vi "Day 8-1.vi"() -> ()   [LabVIEW 2019, in "Day 8.lvlib"]
uses:
  Day 8.lvlib
panel:
  out "Array":string[][](array[string])
  out "disabled index (col)":i32
  out "array type (2D Dbl)":string[][](array[string])
  out "subarray":string[](array[string])
  out "array":string[][](array[string])
  in  "String":string="ecgabfd gfbe dgbeaf aeg gfbda eg bgdcaf efgdca abced eadgb | begf decgfa aeg eg\nebfg bfgdea gaf gf baedgc dafec cfdabg ecfabgd fdgea dbaeg | gaedbc egbf dbgcea dagfebc\ncfadeg ca bacg dfabe dgcbf dbegafc dac afbdgc gcbedf bfcda | fbdac adbef bgcdfae dcagfe\neag cdgfae cbdge ae fcgad eabdfg ecaf gefbadc dgafcb degca | dacbefg fcdage agdcf fedagb\ndga edac gdfbea bgdfec da cfbga dbgec cadgb bdgace dcbfage | acgfb gaecbfd dag gedfab\ncefb fb abcgefd fagbde fcbgae faecg cbadg cbfga bfa agcdef | gbacf agbfc bgcaef baf\nebdacf cbgfae cgdebaf afdcb gabdc df cdf eafd ecabf begdfc | cbdaf gdabc fd cbefda\nge daebc fcagb fdebac gaed ecabg egc gacedb cbdfeg adcfbeg | gec gebdca ebagc adbgcfe\nbgfade gcefbd eafgd fcae cadgf gcf dgcba cfdega cagbdfe cf | cdgeaf agfed cf cf\nabfge ebac acfegbd bc fcged gbfec cfgbad fecabg agbfde fcb | aefgdb cfb egbfca cbfaedg\ndfcbag gda dcafe gcdeb ag ecgdaf edagc bcdaef gcbadfe gaef | gbced dga cbadef fgecda\ncagb adgceb cdb cfgeda egfbd abcefd decag bc cgebd bgedfca | cegbd dfegac dbc befdg\ncbfe bgefdc ceabdfg cf dbgaef gdfbac edcga gcfed dfc fbedg | fgbaed fcd fcegd becf\ndegabf bfg bcgaf gdacf dbfc gecfda gcaeb fagedbc adfgbc bf | egbdfa gbf adfbceg dcfb\ndbfae dfbc ecadg cb cbdea fcebag fgadbec gadebf bec ceabfd | dbfc bgfcead agbedf fdabe\ndafcge ecafbg cegaf egdac abegd cd debfca edc cgfd bfdeagc | dec dc ecd dbgae\nfgabce bfa acbfegd fcegda bfgd acgfd bcaed bfcda bf cbagdf | bf bafgcd bfdg dgbacfe\nfgea gad fcbgaed gdebc afdeb fagcbd cbfeda ag egfdba degab | dgeab badge eacfbdg fdceba\nfabdce cagdb gcb bcefag degba dfagbc dgcf dcfab egfcabd cg | befcda dbagc cbdgfa gcdf\nbe fgaced fdeag badegf fdbea ebdg bea agfbec ebgadcf bcfad | acdfge agbfce debaf dgafe\ncdfbeg bg fegca gdefac cadbf eadbcgf cgb egba gcfbea cagfb | gfaced agfcb cbdfaeg cgfdabe\nfadcebg cgda ebfag adebc fcebdg fadbce gd begcda bdg gedba | dcga fbage dcabef fcebadg\nbfcga adfbgc fbcdage gfedac ab gcfbe cgafd efabgd gab bdca | gcafd cdba gba dfabgc\nbdfae gfa cdgabe egfba fg gfeadc acegb fgcb fbecgad ecafgb | bgeaf agfecbd fga agdceb\ndgab ebfad cdefgb gbefd fab cefabg fegcbda aedcf ba ebadgf | defbag afb gbfead dbefag\ncfabed ecabf cgafdeb bfc fecbgd dcab cb bfeda eagfc adfgeb | fgcae dfbega ebcdfg fabec\neb cbgaef eagcfbd caebd gaedbc badfc abe degac dgeb cgdeaf | aeb gfaebc bceafg abcged\ngdecba ecbdgf def fcbade fd fdcg bgfae gdecb gfbde faegdbc | fbage ecgdbf egdfb dfe\ndc dac egcadbf gadbe cgaebd abgcd geadbf agfced edcb gabfc | agcbefd edbc bacfg cd\ngaebfc gdc cedbg dbeag cefd cd bcfgde cbgfda bcegf dabgecf | bgdea dbgec fecd cfed\nafd dfcbga dcbeagf bfecda egbcdf dagec fa bgfa fdbcg fgadc | egbcdf decga gbfa fa\nfg baefc gafeb dgaf cbgdea afegbd fbg cebgfd gaecdfb dbgae | ebfag dgbae gafd abgedfc\ncbaed gedac cefgbda feba be cadebf gdcefb fcbad bde cdagbf | bcadef cfgdab fdabc feab\ncfbdg fdgce adgcbf fb cbf acfegdb adgebc ebafdc dbacg agbf | fgba fgced ecfdabg bf\nfceabd gfb agfdb deabg beacgf cfdgbae fcdg gf abfdc dfbgca | dbaeg bfdga dgeab dfcg\ngfde facbde dcgbf fg gbf ecafgb cfgdbe ecdfb adcgb ecafbdg | gcdbf fg cfbdg fdeg\nfbgdce bg bacefg decab cbg fecgd egdcfa dbfg egdcb fagdbce | gb dcbea fedbgc fagecb\nabgcef fgbaedc dfaebg cgad ad egadcb abd cgbea bfecd cabde | efbcd abdfeg afbegd ad\nfagecdb bcafg ecadfb fa bagecf cdgba efbdcg befgc fac agfe | bdfcge ecgbf cfedba edagfcb\ndgf fcdbg cegbd fd bfcega daebgf dfca abgcf gafbdc fbeacgd | bcfdg fdg dfg adcf\ndeb cbdgae edfbac dbcgf fbecga gdfcbea bgdec ed ecabg egad | bgcfd faedcb cageb ed\ngecfba dfagc afdbc adbcfg cag cabgdfe fdega cbdg dbacfe cg | afcbdeg dabcf cbafed dcfga\nfeab ae cbgfe agecf bgecda bgecdf eca gfebca fcdbgea cgfad | bgdfec gcfbed eca cbdgaef\nfbaceg edcbaf dba becgd egafb degbfca fbadeg dafg da agebd | fbdega gfebca acebdf gbefa\ndbce gfbec defgb ed efdagc def gfbeca abfgd bgfedc fcbgade | fdbgce ebdfcg cgfbdea efcbgd\nabcdfg fcaegb egf dgcaf bdecf aged bdeacfg ge dgcafe gfcde | acbgfd gcadf cgbdaf gafecb\nfb gbfaed eabgdc abcgef adcbfge dgfac fecb bgf fcbga cageb | acebg cfeabg edgcab adgfbce\nfad ceafdg dcfag fbcadge geadbf deac da gcfea gdcfb efcagb | aegdfb cgadf aefbcg bgdcf\ndagcbf ef dacfg gfdce egf ebdgc dfcgea fabdeg aefc ebdacfg | gdefc dcfag bgdceaf acef\ndbegf eabcgd ebdafg fbdac cbg cefg eagbdfc cdbgf gdfbce cg | eabcdgf gecadbf decgbf gc\ndegf cbefd bfcdeg bfdaec bcage cfgdba fg fcg fbcge cefgdba | fged cfgedab fdgceb efcbd\ncgbdae dbeca bcfdeg fcaged edgca be cbdaf ebd gfbadec egba | cefdgab cdfega bcgeda agcbde\ncdfgea gbedacf gacbf cdb decag db edcabf gabedc dgeb bgdca | bcfag bcgad ecdgfab bd\nebcg cfgbae acgdbef eag agdfc ge edgabf cgefa facbe dacebf | cbgefa agcfd fgcad dfgac\nbeagcf dafcgbe da acd bedcf begacd cdbae cefadg bagd bgcae | da fgbecad bdcef bfdec\ndg acgfebd fagecb bgeadf ebfgc gdb cdbgf dbafc gecd debfgc | egcbf cafbd facbd afbegcd\ngeabd cadefb ec eadgfcb cedag gdbeca dec gfbdae dcfag cbeg | ec bdeafgc cbdafe ebcg\nbe bfade caefgb eab gdbafe bedg agfdb edacfbg gdcabf daefc | acfegb bae fecadgb bgcfea\nbe acdfb cgfae cbe agbe fgeacbd adegcf bcfae bgcefa fgbecd | cfabeg ecb efcdbg ageb\nafbg cfedb dacfgb fgdcb bgfedac cbdage bg acgdf fadceg dgb | cdbgfa fgeadc bafg dfbce\ndebfc efb adgbce ef fbadec dfcbg feac dacgebf aebdc eadgfb | fcdgb efca cbdeaf edbca\ngcbde dgcbf dfc bfcgda df ceadgbf gcabf dbaf gcefab dfcega | adfb egcdb dgbce bdfa\negbdca bgfed baefd cfdgaeb gdefc gcbfed gcfead bg cfgb egb | dcbage cbdgef dgfbe aedbcg\ndceaf fc fcge bgdaec agced dfbea cgeabdf adcfbg fdc egcfad | fedca fadeb dabegc aedfb\nacfbgd efcda cfagd decg de efcgdab eabfc gdaecf dae bedfag | fceda acdef ed cfeba\ndefbcg ge egb eagbdc afdgcb cgbae fcadebg geda dcagb efcba | gdecba abgce gbadc daeg\nafbd fadgce gbfdea fcgedb bf bgf gefda bfedgac bgcea gaebf | bgfaed fdgecb fbgedc bfg\ncbafgd cbdge bc cbd bcef fgbde afgbde fgcbed dgebfca edcga | cb cb acged fdgbec\nacgd dceagf dc bafde fbaceg ced cdfbge fdeca egcabfd cgefa | dc egdcfa afegcd efcgbd\nbgdfac fb aebgc bfde bdecaf bfa aebcf edabfcg cgdeaf daefc | decfa fb baf fcbdea\nbdfegc gebda gecbfa fedbg fed dgfc fabdec dbcagef fd gfcbe | edcfbag dgfeb cdeafb fd\ngbeadf fdcga ecadb bceg ge egd dgebacf beafcd aedgc cgbade | dabec dge begdac dgaebc\nbegc dcgbfa eb dfeag eafgb bae bcgaf gfaebc fbagecd becfad | gabdcfe fdcagb bgcdaf be\neca febdcg fedag ecdaf fcba beagdc fcdeb ca dbefca acebfdg | ebdcgf fdceb gecdab cedfbga\ndecfbga abgdce gefd afd aecdbf gcfeda acgde cafbg fd fadcg | edgf dafbceg egfd cedga\nfaedgbc fbgaec dacb eba geacdb bcgefd ba bdegc eadbg gdaef | dfcbge deabcg bfecadg gfcbaed\negfacbd acdgf gecdab ebacf abcfed eg begf caegf aeg bfgeca | dafbcge cadfg fbace cefdbag\ndgcfbae ac gbfeca badce gcad dfgcbe defab cea acgdbe dbgce | cgdeba egcdb gcad cagd\ndcfg agdfbc caedfgb df bagecf daf gcafb ebcad fdbac agebdf | bdfage fgdbac daf fd\nagefbd agcbfde egafb eg adge fge bfaced egdbcf daefb cabgf | bagef afgbe eg efbcdg\nadfegb caefgb ade ecgd cafed dbfeacg de fgcae fbcda fgadce | dbefgac eafcg gbaefc fedgac\ndbafg ecfga gfbae bae egdbac geabfc gcedfab ebcf eb cagdef | be cbfe bae be\ncfgadbe eca bcfadg ebdgac adgcb ebdca adbfe egcb cadfeg ec | adebgc feabd cae cgdfea\ncaefdg cdfagbe fadbc afd eacbd fd bcadeg cgfba dacfeb bfed | df afcgb fceabdg fda\nedcgaf cfbdag cbfdaeg ec cae bgeafc cdafe abfde decg gdcaf | eca dbcafg aec ce\nfbgae cagef egdbac cg gcdafbe cfbg bgefda gce ceadf gebfac | gadbce cdegba gc cg\nbafgecd bdf ecabfg dgbfe dcefg gbefa bdea bdfcga bd bgfdae | cdfagb cfeabg faebgd fagbe\nafg dfcg fg eacdbg fgadeb cfdgea ecagd fcagebd eacfg bacfe | fg dagecb egdca cfdg\ndac dc fgcd agbecf gcdaef agbed edcabf fgace caged faecdbg | dabge gceaf gdafecb cdafgeb\naefbg egf bagcf afegdc dfgceab begd gafebd eafbd eg fabcde | egadfb feg bgcfa efg\nfa debfg acgfdb eagbc dcebagf cedfbg dafe baf febga eagbfd | af cbfdga dcfgab befcdg\ndb dbfe fdbga cafdg adgceb egbfa dbg bgfdcea ceagbf befagd | afdbge dceabg gdfab fdaegb\nfgeacdb cadg dfg edfga fdagce dg dfaec gebfa cbefgd defabc | geabf dfaec cfdae faegb\nabdce bafcg gdecaf cegba fbcadge adbcfe degb eg bdcgae eag | abdec facbg edgb ebagcd\nbcaef fg dgbcae adegb bafeg feadcgb egbfad fdgb fecagd efg | agfeb fge fdgb eadgb\ndbfage cdab bgcaef ecb cb dgfce dfbce fedbgac deabf beadcf | cbfed dabfe ebadf cefbd\ngcedb ceafdg dcg gecdfb dcfaeb cg egdba befdgac fdceb gcfb | begdc bedag eadgb dfecb\nbf dbcgea eabdfc feb gbfeac fagb becga fcdaebg dcgef gecfb | efbdcag abceg gcdabef gcbef\nged dagfbe eg cgfe bgfacde gedac dceba agcfd cadegf gcfdba | gefc ge ge acegfbd\ngfabed aecdgf ecbag dge gbdae befd bfgad fdcabeg de fagbdc | egbad afdbg dgacef gdafb\ndabfegc gbcad gafd acd da fgbadc ecdabf bfgca fcabge gbdec | gbface fgcab bdgac ebdcg\nafbceg cdgfb gb afcbed dfcbge gbf adfgc fecbgad egdb bcdfe | fedbc cfeabd edbg cfebgd\ncbdae gc gdfc ebgdf gcafbe fbaecdg gbedc ecg fbgecd fdebag | gcedb ebgafc acfgdeb ceg\nbdce efacgd dgfbc ebfgad bcfga gdc fgbedac egdfb dc bfdgce | bagdfec efdgb ecbd fdaegc\nbdgefc fbca bc gfbcae fdcgae gdaeb cbega gcb efagdcb feagc | gcb bacefgd ecdbgf cfab\nfdbe defcbga adf cfgeba gcdae bacef cfadgb df fdeca dcefba | cbegfa degfcab fad acgfbe\ngabfdc ebcfd bacgf da fcgbea aedbfcg gdfa eadcbg cdfba abd | dab dabcf afcgb ad\ngb bfgcae dbgf cadeg bagdc gefadcb gbc acdbef cgabdf dbafc | gb fbdcae afdbgce dabgc\ncfgadbe agecfd ea gedfc edafc fage fbdgce ead aecdbg fabdc | fcbdage cdbage fbadc ae\ndecgbaf edcgba afgd aebgfd da bfeag gfbcae bad cebfd bfeda | ecfdb eagbf efdba eabgdf\ncfdbae dc gbdef fbedag egbfcd gafec edc edacgbf egdcf bdgc | fceag gacfe daegfb bgdcef\ncbgda egdfb agebd cgedfb aed bfgdcea ae agdefb efab facedg | gdcaef aefb faeb begfd\nfdc begdf adecg gfaced cf efac abedfgc cbedag gdbacf fecgd | cdf fbgadc cabgdf acfe\nfedbg gabfe feda gde fcdbg de dbegacf bdfaeg abcdeg cegbfa | bgaef gadebf efgbac gbefa\ndgf fgdbea dg dafcb gdec edcfbga dbegfc gbdcf cfbge gcebfa | bdfgc dg egcfab bcdafge\nceg daecb gcfdea fgacbe ecadbfg eg gbacdf cgabf ebfg ecabg | acgeb bfgca geacdf cge\nge geabf gea abecgf fdabg caedbf egbc cgebafd cbfea agdefc | feabc bcdafe age eg\ngecdba ebdfg gcdef ecf cefadb fgac cf ecgafd cbfgead adgec | dfecg afcg bcfead ecadg\ngd cbfad fdagb cfbeag fabge efabdg aged bdgfec dgf gbfadec | acefgb eabfgc becagf bfgda\nebgc fedabcg fdbgce fdebg eg badgf ebcdf edg adcfeb cfgade | bgefd cbgefd bgefd abfdg\ndgbfc abecfg gcdab fcgdbe dfge cbdfea defbc fgc dabgefc gf | gf dbgecf bafgec cgf\ndegbac fda cdbag eafgbcd df fdbc agfdcb dabfg fbgea fcgade | fd bdceafg fdagbce df\ncedaf fgeabc egdbf gbaedcf aeg cgda dfaeg cfdbea fagdce ga | febadc gefad bfacde gae\ngea ebfgdc bcae cgafd abecfgd gbced ea gbdeaf dcgae gebcda | efgdab fcegdb cbgade acged\ncdabgef gb fceag fgb bfdgac gbcfa cbadfe dfcegb fbdca bgda | bg cbgfa dcfgeb afcgb\nfcbage adefc gceda bdegca cbeag dgeb efacdgb cfbgda adg dg | gad gabced gebd dg\necbdga gedbf dafeg faecbdg eacfg dbaf ad dbfcge gda dfbeag | ad gfbcde dgfea aecfg\nagfbde begfca bca baegc bc bcef ecdgbfa adegc bgaef acbfdg | fdbcag baecg cgdbaf bcdagf\nbeafc badfc daecfb fd fad fdec badefg cbdag fbecgad gecfab | dcfe cbgeaf gdcfabe agdbc\ncaedgbf fcgead ca gbadf abcd adcfbg fegbc dfaebg gfbac agc | fcgeda dbac afcgb dafebg\ngdfeb gdbafe bc ecb ebfagdc bgfce gfeca fdcbge aebdcf bcdg | cdfbeg gdbfe gefcb dbcafe\ngfbca gcdfe dbafgc cafgbe eacfbgd cdb agdb db cgdbf ecdbaf | adfcbe abdgfc cdb fcabed\nbcdaf fbed edbac cdaegf ed dbgaecf edc ebgac dbagfc fdbace | cbgae efdb gcdafe gbafedc\ncdfba cbdfae cfga bafdgc aedfgbc dbgef dag adgfb bdaegc ag | ebacgd adfgcb bdaefc gfac\ncaefd ce abfdc egcbdf cfe fgaced bdgfea gcae fadcbge eagfd | fcdae fgecad ec cbefgd\neafbd deb aefdg bd aecfbg bdcf abcfe gebcdaf agdbec bcaedf | dbcfae abfecd efabcd cbafe\nbdafeg efg gfcdae bagfd dfacgb ef dgfecba befa efbdg dbceg | fe gadbf aebfdg afeb\ncgbef ceb bfdgcae gedbac acgfbe be gceafd eacfg fcdgb fbea | abcedg dcgefa be fcegadb\ngacb gfbaedc fagdc baf gadcef bfcdea fgebd gfabd cfdgba ba | baf cadfg gbfad fab\ngafce df cbdfge gfd gdecb gecdf fdeb cadbeg agdbcf abgdcef | cgfea abgcde decgf fgcdbea\negdbf cbfgde aed befa gfdbae ea abcgd edfcga bcaegdf agdbe | bfae cagbfde cbgda gedcaf\neb dfbacge dbgae becafg abe gadfb cdega cedagb ecfgad debc | cfgeda fagedc afdbg fdcega\nefcba becagd gafcdbe eafdbg dagbcf agfbd gefd de bfaed deb | fabce bgaedc ceadbg bed\ncbaedf fdgebca gdbe dabce eag ge bacge bagcf decfga bgecda | defgabc bceagd aeg gbacf\ndgeabf aefgcdb ad bcfae bdacf dacg bgfdc ebfdgc gfdbac abd | dcga adgc decfbg bafce\nfgcba cbdfeag dagfb dcgbaf dcaegb ecbafg bdg bd fcbd faegd | bgdaec feadg cbdage dcgafb\nbdc dcfgeb ebgca bdea bdcga abfecg gdcaf bd aecdbfg aebgdc | bade bdecgf bdc cbadg\nbcdaeg facgbd caedfb aefdb dgfbe eba ae dcegfab fcea fbcad | cbafed baecdf ae ceabfd\nefcbg egd dg cabgef bfdceag fgcbde fdcea gdfb dgebca dfcge | fdgb gd fbgd deg\ncbgdfa ebgcfa abdge bdeca efcgbad cd fbedac abecf adc edcf | agebd gfabedc dabfegc abfce\nedg abdgce gcefb dcbge dgabfe gcdab de cdebfga cdae fdabcg | gbdafc agcdb dgfceab bafgdec\nacdb dgbfec eagfcdb dafbec cae ebdfc ca gfaed acdef gfebac | defac begdfc daegf fdeacb\ncgedf gfadce debgcf fedagcb aefbc bcdagf db ebfcd bfd begd | db cgfde dbefc gedcfb\nafcbegd dcfge edgbf bdg fabd dabfeg gaebdc abgecf gfeab db | debacg gfbaec fadbegc afcgbe\nfcbg cdegf ecdga eacdfb befdg dcf fc dfegba dbfgce agdfcbe | dcf adcge fbcg dgaefbc\nbcfea fcbead ecd cgeafb aebcgd bfed bcgedfa de cadfg fedac | de egadfbc debf bfagec\nefcdabg afecbd defba cabfd ebca cgdaf dfabeg bc efcdbg fbc | bgdefc afcgebd gdefcb efabgd\nedbaf agfbcde gbfcae ag dega aefcdb dfbega dfgbc afdgb bag | dagefb ga decbfa aecbgf\ncbdg aegbcfd badce dgaebf abdcfe gad cgeda gd fcage ceagbd | fdcaeb dbeca beafdc bdace\ndecb dagfe dcgbafe fecbda acfdb adfbcg agefbc fec ec faced | fcadeb cdagfb agbfce gcfdba\nacdbef dgca gbfae agecfdb ebdcg bda bgeda gedbfc ad bcadge | cgdbe cdag dcga efdcgab\ngc efbdg eadcf ebcafg adecgf gfdbaec gcf gcda dcgfe dcbaef | gc acedbf fcead gdca\nbfgce dabfg ecdf cebgfa dfegb ed deb fecbgda becgda cfbedg | cdgbefa ebd gafdb cdgefba\nce gecb ecd debaf ecdfb dcfega dagcbef fbgcd bdcgaf dcgfeb | dec dfbec agcfed bedfa\ncgbfd gb dcafg gadb gbfcea bcfdeag fcbde fbg gcbfad agdfec | dcfgab bfgdc dfaceg dfgac\nbgacef cdagf bgdcae gd dag dbagfc fecagbd fdbg cfead agbfc | gfcba adgcf facgb gd\nefdc adbgc gec acfgde feadg gbecaf fbdgae agdec daefbgc ce | ec cedf cge bdfagce\naecdbg cabfe acfgeb bcefda fgac fdgeb afdcbge bcg cebfg gc | gcbfae febcda facg baefcg\ndgbafce gfacdb gecb dcaefg gfaeb egf gebacf bdefa bgcaf eg | abfge fgabe fge deagfc\nceafdb dcbega afd gdbeaf fdgea fgeac gbade cbfadeg fd dfbg | adbcge gdcfeab afd fd\ndacegf ed dfcbg cfgea dcfge fcgdbae acgbef ced eagd abefcd | dfbeac fgcdb geda dbfgc\negbcdf ecbdga afegc aefdbgc dgeca dge dg dcfbae dgab cdbea | gcead eabdcf gdeac cfadbe\ngca fceagd fdgbc ga fecab fgcabed bgcaf cdbfge adbg acdfgb | agdb bfadcg bfgac gbfca\nacgdeb baefd fa gdfa bgdea bdcfe fdagebc fdgbea ecfgba fab | adbecg agcbed febagc feagcdb\nfedagc dcfge ef bgdcf gdceba egf fead edcag gfbaec fdgaebc | cgade aecfdg efg eadf\ndbagf gcdefab fc badfc cbaed gfadbe dgfc gfbcad gaebfc bcf | cfb cdbea bdagf fc\nbae be gcadeb dbge dgebacf eagcd geabc fbcga eagfdc edbafc | gcabf ecdfbag afbcg cbgfa\nbd gdbcf cbfegd cfbeag febdagc fbd fcgeb decb afgbed dfgac | cbefg eadcbfg cbegfad egdfcb\nfebacg dega cegfd cefda ae agebcfd abcdf eca defacg ecgfbd | badcf cae bdcefg acedf\ngeabcd gdbcfa gaedc cbeagf bdgeacf gdefc bdacg ae adbe cae | gcebad agfbdc gefbcad ea\nfa bfdacge adecgb eacf bdfgac gfdbe aegdc egacfd gadfe fga | gedfb egfbd efagd dagfbc\ngcdb dg beagdf feacg cebgdfa afbcd adcgf dbfcga ebfdac agd | gd acdfg dcbaf gacfe\naefgbd cgfdb gfdea eabfgc dcgfe cfe ceda gdcaef ce fdeabgc | bdcgf edgaf cbdfg egfbda\nfacegb cfdabeg bd cedgbf adcfeb cfabe cdb eadb cgdfa dfbca | dfbca eadb adecbgf bdc\nbacfeg agfcdeb acegf gfcade ecagbd fdbag afegd cdfe ed edg | dfce egd degaf dagfb\ndf gdfcea efbadg cegafbd eacfd fad cedbga dgaec dfcg fbcea | caedg dgafbe edgac df\nbfdac cdbgfa cefbgd bfag afgbdec cdgafe cbfdg acf ecbda fa | dgcfae af cabfd beadc\nbefgd dea ecab baefcd gfbcad ea bafcd dbcgefa afebd cadfeg | gfbadc eda cadgfb eda\ngf cgadb gebf becfdga gaefcd febac gcbaf cbfdea bfgeac fag | fg afcbg efbg afg\nba aebg gafdceb bca bdacg dagcf fcbdae gcbed cadebg bgcefd | dcagf gdabc afgcd edcfgb\nde dbec bfaecdg gdfeca fegcb edg dbgaf fceabg febcgd bgdef | afdbg adbfg debfgc bdgfa\nafbced adebfg efagdbc caebf afgec ecgb ega eg fgdac acegfb | aedgbf cbge egbfda badfgec\nfg gbfcdea eafbcd fdaeb cdage egf agdefb fdcbge efgda fgab | deacg cdage gedca adfeb\ngde gbdc dg fdgec dfaegb fedca bcgefd fbeacg gadecbf fcbeg | cgfabe edcgf fgeabdc cbefg\nbefcdg agbcef fcbdeag gdfae bdecf eab fcdeab ab efbad bcad | cfgeba befda aefgd degbcfa\nabcef dbfaegc aefcg dcgbae fbcg efgacb cg cdabfe gec dfeag | dgfae gdefa agcbde afbced\ndgf fcbega afdbeg fgabe dg efadg bged adfbceg agbcfd fedca | aefgb begd fceda debg\ncdgaeb ba befgdca defbc gdecaf bae gabc afgdeb gedac decab | fbecd bae gdecfa edcba\nebagfd dfg dcbaeg dgbceaf gf gacdf fcade gacbd gcfb fbagcd | adgfc acbgd edbagf degabc\ngba eagbcf gb gbacf dacgebf bceg gcafed acfeg acbfd adegfb | abfcdeg dbcfage faecg afebgc"
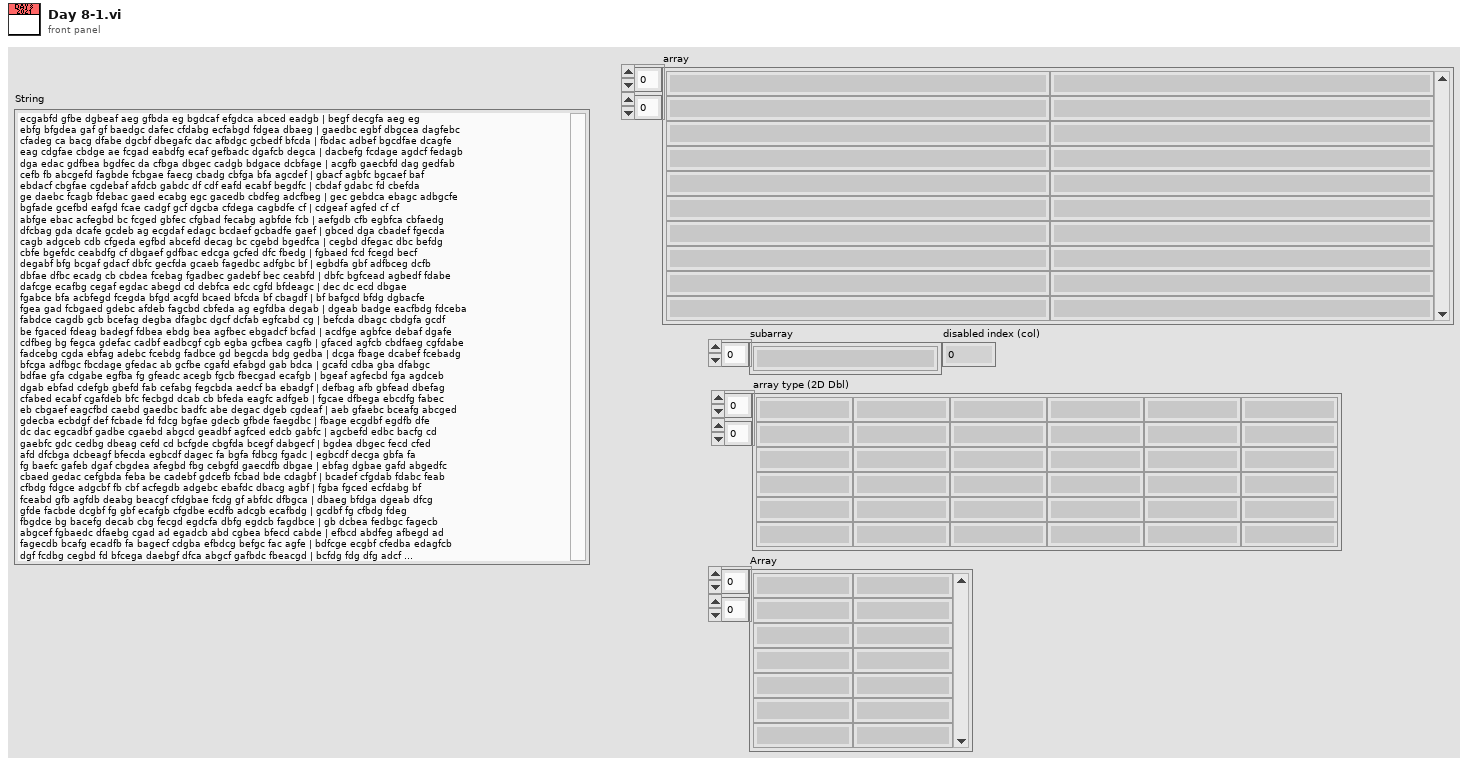
[diagram p1: front panel]
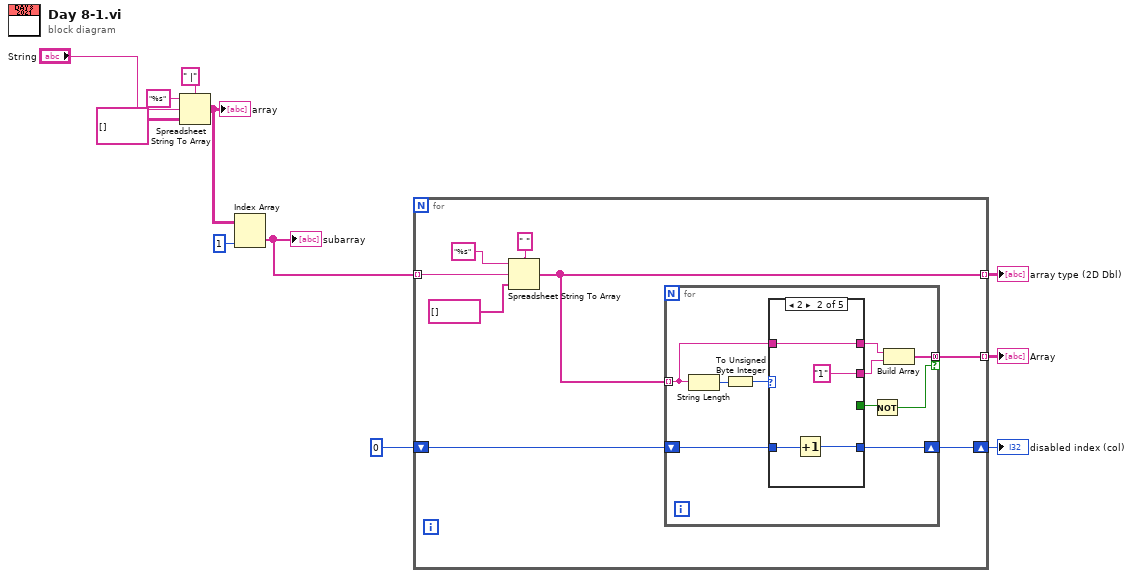
[diagram p0: block diagram]
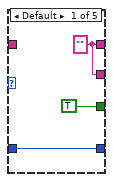
[diagram p2: hidden frame]
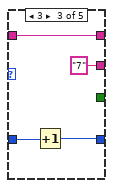
[diagram p3: hidden frame]
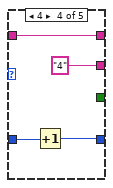
[diagram p4: hidden frame]
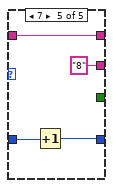
[diagram p5: hidden frame]
diagram:
  n1 = Spreadsheet String To Array(delimiter (Tab)=" |", format string="%s", spreadsheet string="String", array type (2D Dbl)=string[][] []) -> (array=w7:string[][])
  "array" <- w7
  n2 = Index Array(array=w7, index (col)=1 ("disabled index (col)")) -> (element=w5:string[])  [unwired: 1 in]
  "subarray" <- w5
  n3 = for {
    tunnel: w5 -> [w19] mode=indexing
    tunnel: [w15] -> w4 mode=indexing
    shift-right: [w13] -> w2
    shift-left: 0 ("disabled index (col)") -> [w14]
    tunnel: [w12] -> w1 mode=indexing
    n4 = Spreadsheet String To Array(delimiter (Tab)=" ", format string="%s", spreadsheet string=w19, array type (2D Dbl)=string[] []) -> (array=w15:string[])
    n5 = for {
      tunnel: w15 -> [w25] mode=indexing
      shift-right: [w26] -> w13
      shift-left: w14 -> [w27]
      tunnel: [w22] -> w12 mode=concatenating if=w20
      n6 = String Length(string=w25) -> (length=w29:i32)
      n7 = To Unsigned Byte Integer(number=w29) -> (unsigned 8bit integer=w28:u8)
      n8 = case shown="2" w28 {
        tunnel: w27 -> [w32 w36 w40 w44 w48]
        tunnel: [w32 w35 w39 w43 w47] -> w26
        tunnel: w25 -> [_ w34 w38 w42 w46]
        tunnel: [w31 w34 w38 w42 w46] -> w24
        tunnel: [w31 "1" "7" "4" ("format string") "8" ("format string")] -> w23
        tunnel: [TRUE _ _ _ _] -> w21
        frame Default {
          w31 = "" ("format string")
        }
        frame 2 {
          n9 = Increment(x=w36) -> (x+1=w35:i32)
        }
        frame 3 {
          n10 = Increment(x=w40) -> (x+1=w39:i32)
        }
        frame 4 {
          n11 = Increment(x=w44) -> (x+1=w43:i32)
        }
        frame 7 {
          n12 = Increment(x=w48) -> (x+1=w47:i32)
        }
      }
      n13 = Not(x=w21) -> (.not. x?=w20:bool)
      n14 = Build Array(w24, w23) -> (w22:string[])
    }
  }
  "array type (2D Dbl)" <- w4
  "disabled index (col)" <- w2
  "Array" <- w1
